vi "NIPKG Info to MCL Table.vi"(11 "NIPKG Array":cluster{i32, "package attributes":T1}[](array[cluster])) -> (3 "MCL Display Table":string[][](array[string]))   [LabVIEW 2017]
doc: "Converts a list of NIPKGs into a 2D string array for display in an MCL."
uses:
  <vilib>/National Instruments/NIPM API (Beta)/_support/package attributes.ctl
  <vilib>/National Instruments/NIPM API (Beta)/NIPM_API.lvlib
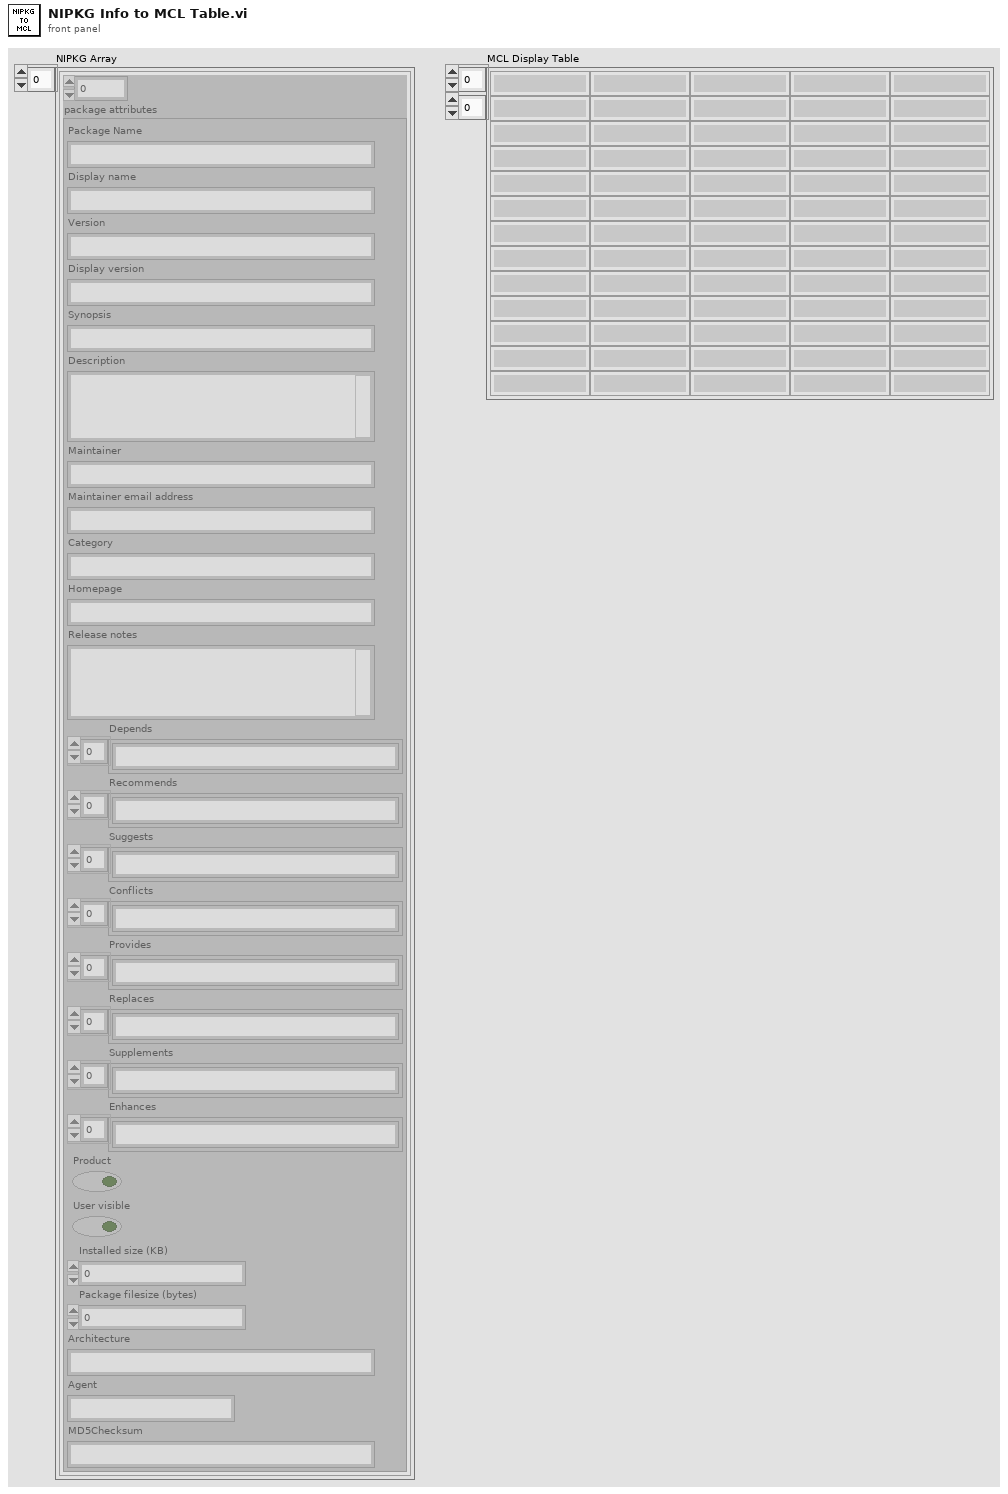
[diagram p1: front panel]
types:
  T1 = typedef "NIPM_API.lvlib/package attributes.ctl" = cluster{"Package Name":string, "Display name":string, "Version":string, "Display version":string, "Synopsis":string, "Description":string, "Maintainer":string, "Maintainer email address":string, "Category":string, "Homepage":string, "Release notes":string, "Depends":string[], "Recommends":string[], "Suggests":string[], "Conflicts":string[], "Provides":string[], "Replaces":string[], "Supplements":string[], "Enhances":string[], "Product":bool, "User visible":bool, "Installed size (KB)":u64, "Package filesize (bytes)":u64, "Architecture":string, "Agent":string, "MD5Checksum":string}
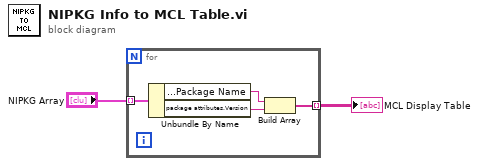
[diagram p0: block diagram]
diagram:
  n1 = for {
    tunnel: "NIPKG Array" -> [w6] mode=indexing
    tunnel: [w3] -> w2 mode=indexing
    n2 = Unbundle By Name(w6) -> ("package attributes.Package Name"=w5:string, "package attributes.Version"=w4:string)
    n3 = Build Array(w5, w4) -> (w3:string[])
  }
  "MCL Display Table" <- w2
